vi "get_http_version_and_status_string_line_for_headers.vi"(8 "error in (no error)":errorcluster, 9 "response_version":string, 10 "status_code":u16) -> (0 "error out":errorcluster, 2 "http version and status string":string)   [LabVIEW 2020, in "HTTP Client reqwest.lvclass"]
uses:
  HTTP Client reqwest.lvclass
  HTTP Client reqwest.lvclass/HTTP Client reqwest.ctl
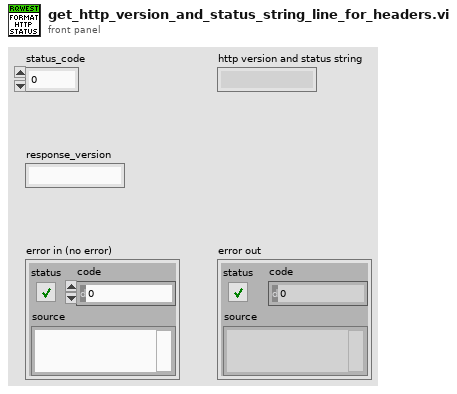
[diagram p1: front panel]
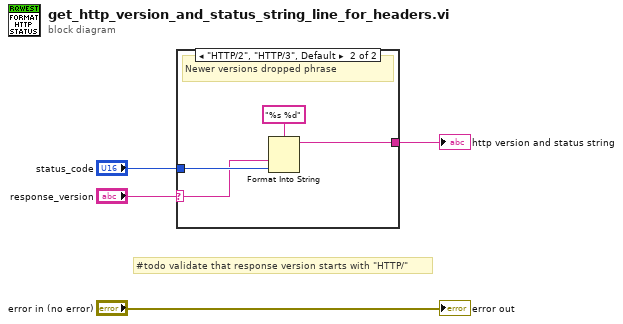
[diagram p0: block diagram]
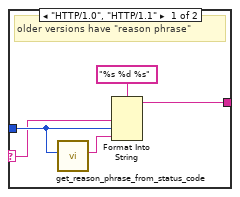
[diagram p2: hidden frame]
diagram:
  # "#todo validate that response version starts with \"HTTP/\""
  n1 = case shown="\"HTTP/2\", \"HTTP/3\", Default" "response_version" {
    selector: "response_version" -> [w5 w10]
    tunnel: [w8 w12] -> w3
    tunnel: "status_code" -> [w7 w11]
    frame "HTTP/1.0", "HTTP/1.1" {
      # "older versions have \"reason phrase\""
      n2 = call "get_reason_phrase_from_status_code.vi"("status_code"=w7) -> ("reason_phrase"=w6:string)  [unwired: 9 in, 1 out]
      n3 = Format Into String(format string="%s %d %s", w5, w7, w6) -> (resulting string=w8:string)  [unwired: 2 in, 1 out]
    }
    frame "HTTP/2", "HTTP/3", Default {
      # "Newer versions dropped phrase"
      n4 = Format Into String(format string="%s %d", w10, w11) -> (resulting string=w12:string)  [unwired: 2 in, 1 out]
    }
  }
  "http version and status string" <- w3
  "error out" <- "error in (no error)"
